vi "XNET.CAN.BusMonitor.CreateInstance.vi"(7 "Listening Port (0 = auto)":i32, 8 "error in (no error)":errorcluster, 10 "Name":string, 11 "IP":string) -> (0 "error out":errorcluster, 3 "gRPC Container out":refnum<class "XNET.CAN.BusMonitor.API.lvclass">)   [LabVIEW 2025, in "XNET.CAN.BusMonitor.API.lvlib" / "XNET.CAN.BusMonitor.API.lvclass"]
uses:
  XNET.CAN.BusMonitor.API.lvclass
  xnet_can_bus_monitor_api_server/RPC Service/NI_XNET_CAN_Bus_Monitor_API/NI_XNET_CAN_Bus_Monitor_API.lvclass
  C:/Program Files/National Instruments/LabVIEW 2025/vi.lib/gRPC/LabVIEW gRPC Servicer/ServiceBase/ServiceBase.lvclass
  XNET.CAN.BusMonitor.API.lvclass/XNET.CAN.BusMonitor.API.ctl
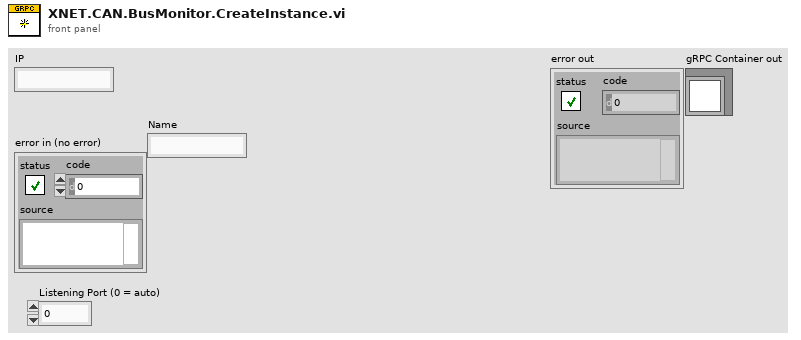
[diagram p1: front panel]
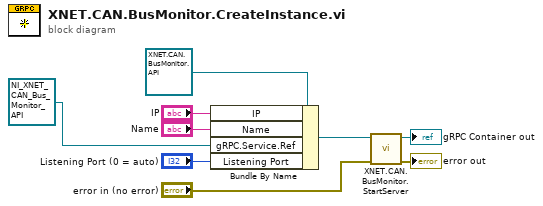
[diagram p0: block diagram]
diagram:
  n1 = Bundle By Name(cluster=refnum<class "XNET.CAN.BusMonitor.API.lvclass"> refnum ("gRPC Container.lvclass"), "IP"="IP", "Name"="Name", "gRPC.Service.Ref"=refnum<class "NI_XNET_CAN_Bus_Monitor_API.lvclass"> refnum ("xnet_can_bus_monitor_api_server.lvlib:NI_XNET_CAN_Bus_Monitor_API.lvclass"), "Listening Port"="Listening Port (0 = auto)") -> (w7:refnum<class "XNET.CAN.BusMonitor.API.lvclass">)
  n2 = call-dynamic "XNET.CAN.BusMonitor.StartServer.vi"("error in (no error)"="error in (no error)", "gRPC Container in"=w7) -> ("error out"=→"error out":errorcluster, "gRPC Container out"=→"gRPC Container out":refnum<class "XNET.CAN.BusMonitor.API.lvclass">)  [unwired: 8 in]
